vi "F Dwf Analog Impedance Status.vi"(8 "error in (no error)":errorcluster, 10 "psts":string, 11 "hdwf":i32) -> (0 "error out":errorcluster, 2 "psts out":string, 3 "function return":i32)   [LabVIEW 2021, in "Olasdwf.lvlib"]
doc: "DWFAPI int FDwfAnalogImpedanceConfigure(HDWF hdwf, int fStart); DWFAPI int FDwfAnalogImpedanceStatus(HDWF hdwf, DwfState *psts);"
uses:
  Olasdwf.lvlib
  Windows/System32/dwf.dll
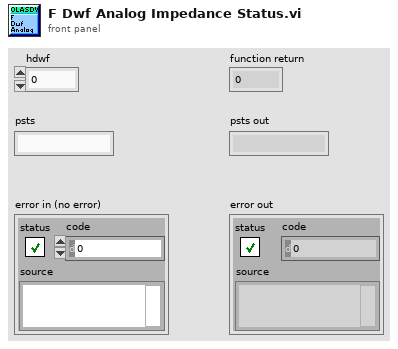
[diagram p1: front panel]
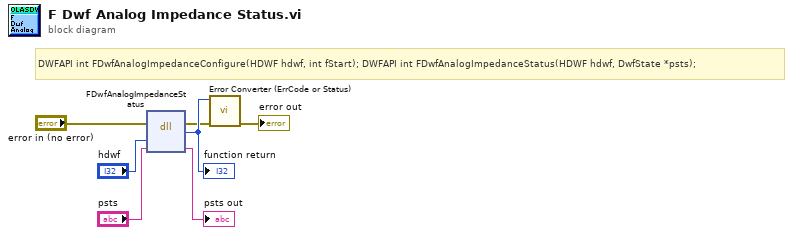
[diagram p0: block diagram]
diagram:
  # "DWFAPI int FDwfAnalogImpedanceConfigure(HDWF hdwf, int fStart); DWFAPI int FDwfAnalogImpedanceStatus(HDWF hdwf, DwfState *psts);"
  n1 = dll-call lib="/Windows/System32/dwf.*" fn="FDwfAnalogImpedanceStatus"(error in="error in (no error)", "hdwf"="hdwf", "psts"="psts") -> (error out=w2:errorcluster, w7:i32, "psts"=→"psts out":string)  [unwired: 3 in, 1 out]
  "function return" <- w7
  n2 = call "Error Converter (ErrCode or Status).vi"("error in (no error)"=w2, "error code"=w7) -> ("error out"=→"error out":errorcluster)  [unwired: 9 in]
